vi "19572_press_START_button.vi"(8 "error in (no error)":errorcluster, 11 "task/channels in":refnum<k21>) -> (0 "error out":errorcluster, 3 "task out":refnum<k21>)   [LabVIEW 2015]
uses:
  <vilib>/DAQmx/write.llb/DAQmx Write (Digital 1D Bool 1Chan 1Samp).vi
  <vilib>/DAQmx/miscellaneous.llb/DAQmx Fill In Error Info.vi
panel:
  # "Press START button on CHROMA 19572"
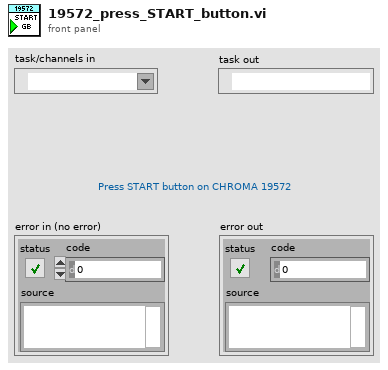
[diagram p1: front panel]
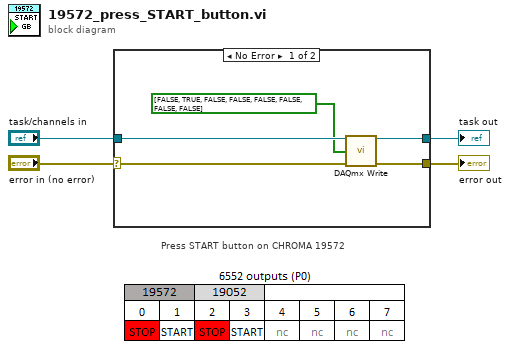
[diagram p0: block diagram]
diagram:
  # "Press START button on CHROMA 19572"
  n1 = case shown="No Error" "error in (no error)" {
    selector: "error in (no error)" -> [w5 w11]
    tunnel: [w9 w11] -> w4
    tunnel: [w8 w10] -> w3
    tunnel: "task/channels in" -> [w7 w10]
    frame No Error {
      n2 = call-poly <vilib>:"DAQmx Write.vi"("task/channels in"=w7, "data"=bool[] [FALSE, TRUE, FALSE, FALSE, FALSE, FALSE, FALSE, FALSE], "error in"=w5) -> ("task out"=w8:refnum<k21>, "error out"=w9:errorcluster)  [unwired: 10 in, 1 out]
    }
    frame Error {
    }
  }
  "error out" <- w4
  "task out" <- w3
